vi "Intan_SamplingPeriod.vi"(0 "VISA resource name":refnum<visa-resource-name>="COM1", 1 "Desired Fs (Hz)":u16, 2 "error in":errorcluster) -> (3 "VISA resource name out":refnum<visa-resource-name>, 4 "FS actual (Hz)":i32, 5 "Actual Sampling Frequency (Hz)":string, 6 "error out":errorcluster)   [LabVIEW 2017]
doc: "use this VI to set the sampling rate (number samples/s/channel). Specify the rate in Hz. \nIn effect, this sets the intervalTimer object on the Teensyduino to precisely time ADC conversions. \nConversion time for 32 channels occurs in tens of microseconds typically. However, ther serial.write() commands typically take 2-6 ms, so the maximum sample rate expected is ~ 100 Hz."
panel:
  out "ack string":string
  out "Teensy fs string written":string
  in  "Teensy event char":string="m"
  # "ADC Sampilng"
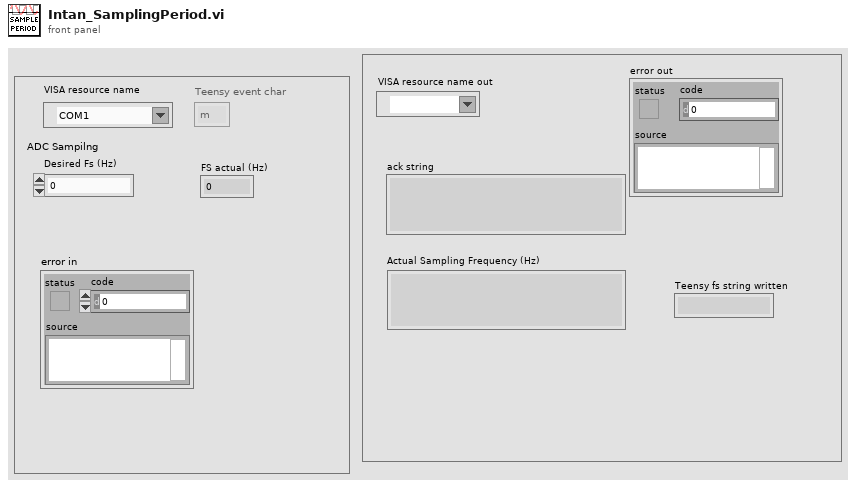
[diagram p1: front panel]
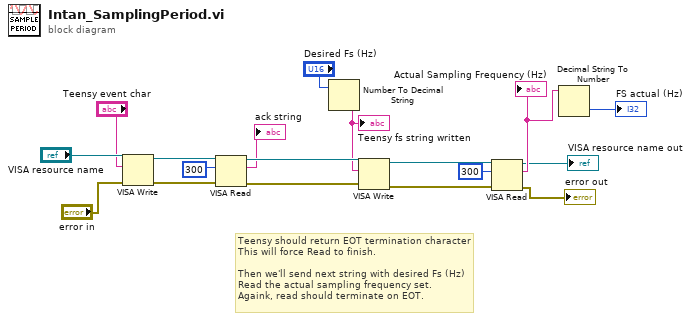
[diagram p0: block diagram]
diagram:
  # "Teensy should return EOT termination character \nThis will force Read to finish.\n\nThen we'll send next string with desired Fs (Hz)\nRead the actual sampling frequency set.\nAgaink, read should terminate on EOT."
  n1 = VISA Write(VISA resource name="VISA resource name", write buffer="Teensy event char", error in (no error)="error in") -> (VISA resource name out=w9:refnum<visa-resource-name>, error out=w8:errorcluster)  [unwired: 1 out]
  n2 = VISA Read(VISA resource name=w9, byte count=u32 300, error in (no error)=w8) -> (VISA resource name out=w16:refnum<visa-resource-name>, read buffer=→"ack string":string, error out=w15:errorcluster)  [unwired: 1 out]
  n3 = Number To Decimal String(number="Desired Fs (Hz)") -> (decimal integer string=w12:string)  [unwired: 1 in]
  "Teensy fs string written" <- w12
  n4 = VISA Write(VISA resource name=w16, write buffer=w12, error in (no error)=w15) -> (VISA resource name out=w5:refnum<visa-resource-name>, error out=w4:errorcluster)  [unwired: 1 out]
  n5 = VISA Read(VISA resource name=w5, byte count=u32 300, error in (no error)=w4) -> (VISA resource name out=→"VISA resource name out":refnum<visa-resource-name>, read buffer=w11:string, error out=→"error out":errorcluster)  [unwired: 1 out]
  "Actual Sampling Frequency (Hz)" <- w11
  n6 = Decimal String To Number(string=w11) -> (number=→"FS actual (Hz)":i32)  [unwired: 2 in, 1 out]
